vi "Configure.vi"(0 "Display State In":T2 {"Time_data" format="%<%.3X>T"}, 1 "Channel Tags":string[](array[string]), 2 "Y-Axis Labels":string[](array[string]), 5 "Variable Tags":string[](array[string]), 9 "Container State":T3, 11 "error in (no error)":errorcluster, 12 "Plot Details":T1(array[cluster]), 13 "history":u16) -> (4 "Display State Out":T2 {"Time_data" format="%<%.3X>T"}, 15 "error out":errorcluster)   [LabVIEW 2016, in "2D Buffer Display.xctl"]
uses:
  2D Buffer Display.xctl
  <vilib>/_xctls/Container State.ctl
  Graph_State.ctl
  <vilib>/_xctls/XControlSupport.lvlib
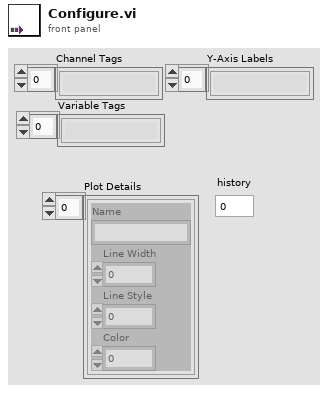
[diagram p1: front panel]
types:
  T1 = cluster{"Name":string, "Line Width":u8, "Line Style":u8, "Color":u32}[]
  T2 = typedef "2D Buffer Display.xctl/Graph_State.ctl" = cluster{"History":u16, "Time_data":timestamp[], "Data_Out":sgl[][][], "Channels":bool[], "Variable":bool[], "Variable Tags":string[], "Channel Tags":string[], "Plot Details":cluster{"Name":string, "Line Width":u8, "Line Style":u8, "Color":u32}[], "Y-Axis Labels":string[], "Avg Data":cluster{"mean":dbl, "standard deviation":dbl}[][]}
  T3 = typedef "XControlSupport.lvlib/Container State.ctl" = cluster{"Indicator?":bool, "Run Mode?":bool, " Refnum":refnum<vi>}
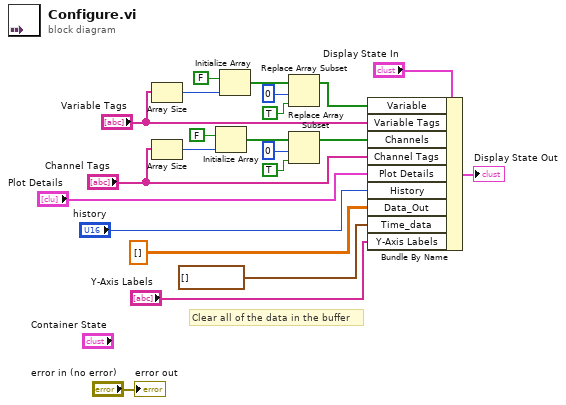
[diagram p0: block diagram]
diagram:
  # "Clear all of the data in the buffer"
  n1 = Array Size(array="Variable Tags") -> (size(s)=w15:i32)
  n2 = Array Size(array="Channel Tags") -> (size(s)=w4:i32)
  n3 = Initialize Array(FALSE, w4) -> (w5:bool[])
  n4 = Initialize Array(FALSE, w15) -> (w14:bool[])
  n5 = Replace Array Subset(array=w14, new element=TRUE, index=0) -> (w9:bool[])
  n6 = Replace Array Subset(array=w5, new element=TRUE, index=0) -> (w2:bool[])
  n7 = Bundle By Name(cluster="Display State In", "Variable"=w9, "Variable Tags"="Variable Tags", "Channels"=w2, "Channel Tags"="Channel Tags", "Plot Details"="Plot Details", "History"="history", "Data_Out"=sgl[][][] [], "Time_data"=timestamp[] [], "Y-Axis Labels"="Y-Axis Labels") -> (→"Display State Out":T2)
  "error out" <- "error in (no error)"
